vi "RobotDriveGlobal.vi"() -> ()   [LabVIEW 2015]
uses:
  Advanced Drive VIs/RobotDrive Type Def.ctl
  <vilib>/Rock Robotics/WPI/MotorControl/WPI_MotorControlDeviceRef.ctl
  <vilib>/Rock Robotics/WPI/MotorControl/WPI_MotorControlType.ctl
  <vilib>/Rock Robotics/SystemInterfaces/DIO/FPGA_DIOPWMChannel.ctl
  <vilib>/Rock Robotics/WPI/PWM/WPI_PWMDeadband.ctl
  <vilib>/Rock Robotics/WPI/CAN/Jaguar/SubVIs/WPI_CANJaguar_ControlMode.ctl
  <vilib>/Rock Robotics/WPI/CAN/TalonSRX/WPI_CANTalonSRX_APIControlMode.ctl
  Advanced Drive VIs/Drive Motor Settings.ctl
  LED Lights/Error Type Defs/Drive Error Type Def.ctl
panel:
  out "RobotDrive Errors":T1
  in  "Turn Damp":dbl
  out "RobotDriveRef":T2={"RobotDriveDevRef"={"DevStatus"={"status"=FALSE, "code"=0, "source"=""}, "Motors[]"=[], "Square Inputs"=FALSE, "Max Output"=0.0}, "Control Mode"=enum."Percent VBus", "Motor Settings"={"Wheel Radius"=0.0, "Encoder Ticks Per Rev"=0.0, "Gear Ratio"=0.0, "ClimbRev"=0.0}, "Default Control Mode"=enum."Unchanged / Invalid"}
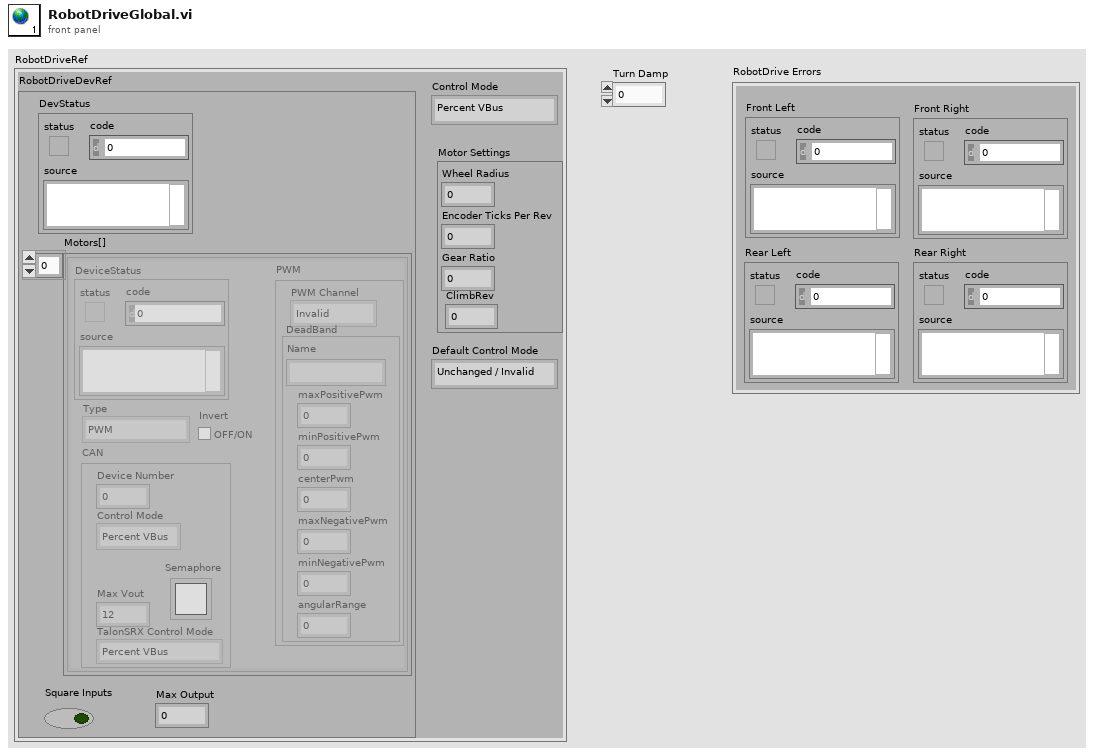
[diagram p1: front panel]
types:
  T1 = typedef "Drive Error Type Def.ctl" = cluster{"Front Left":errorcluster, "Front Right":errorcluster, "Rear Left":errorcluster, "Rear Right":errorcluster}
  T2 = typedef "RobotDrive Type Def.ctl" = cluster{"RobotDriveDevRef":cluster{"DevStatus":errorcluster, "Motors[]":T3[], "Square Inputs":bool, "Max Output":dbl}, "Control Mode":T9, "Motor Settings":T10, "Default Control Mode":T9}
  T3 = typedef "WPI_MotorControlDeviceRef.ctl" = cluster{"DeviceStatus":errorcluster, "Type":T4, "PWM":cluster{"PWM Channel":T5, "DeadBand":T6}, "CAN":cluster{"Device Number":u8, "Control Mode":T7, "Semaphore":T8, "Max Vout":dbl, "TalonSRX Control Mode":T9}, "Invert":bool}
  T4 = typedef "WPI_MotorControlType.ctl" = enum16{"PWM", "CAN", "CANTalonSRX"}
  T5 = typedef "FPGA_DIOPWMChannel.ctl" = enum8{"PWM 0", "PWM 1", "PWM 2", "PWM 3", "PWM 4", "PWM 5", "PWM 6", "PWM 7", "PWM 8", "PWM 9", "PWM MXP 0", "PWM MXP 1", "PWM MXP 2", "PWM MXP 3", "PWM MXP 4", "PWM MXP 5", "PWM MXP 6", "PWM MXP 7", "PWM MXP 8", "PWM MXP 9", "Invalid"}
  T6 = typedef "WPI_PWMDeadband.ctl" = cluster{"Name":string, "maxPositivePwm":i32, "minPositivePwm":i32, "centerPwm":i32, "maxNegativePwm":i32, "minNegativePwm":i32, "angularRange":u16}
  T7 = typedef "WPI_CANJaguar_ControlMode.ctl" = enum8{"Percent VBus", "Current", "Speed", "Position", "Voltage"}
  T8 = typedef "Semaphore RefNum" = refnum<k1>
  T9 = typedef "WPI_CANTalonSRX_APIControlMode.ctl" = enum8{"Percent VBus", "Speed", "Position", "Slave", "Unchanged / Invalid", "Voltage Compensation", "Current", "Motion Profile"}
  T10 = typedef "Drive Motor Settings.ctl" = cluster{"Wheel Radius":dbl, "Encoder Ticks Per Rev":dbl, "Gear Ratio":dbl, "ClimbRev":dbl}
diagram:
